vi "readMATFIle2.vi"(11 "selected path":path) -> (0 "dt2":dbl[](array[numeric]), 1 "Graph":cluster{dbl, dbl, "Magnitude":dbl[]}[](graph), 2 "Array":T2(array[cluster]), 3 "Title":string, 4 "npts":dbl, 5 "fsampling":dbl, 6 "tfun":dbl)   [LabVIEW 2024]
uses:
  Subs/miDataType.ctl
panel:
  out "text translated":string
  out "Left":string
  # "time chan    spect    sonogram"
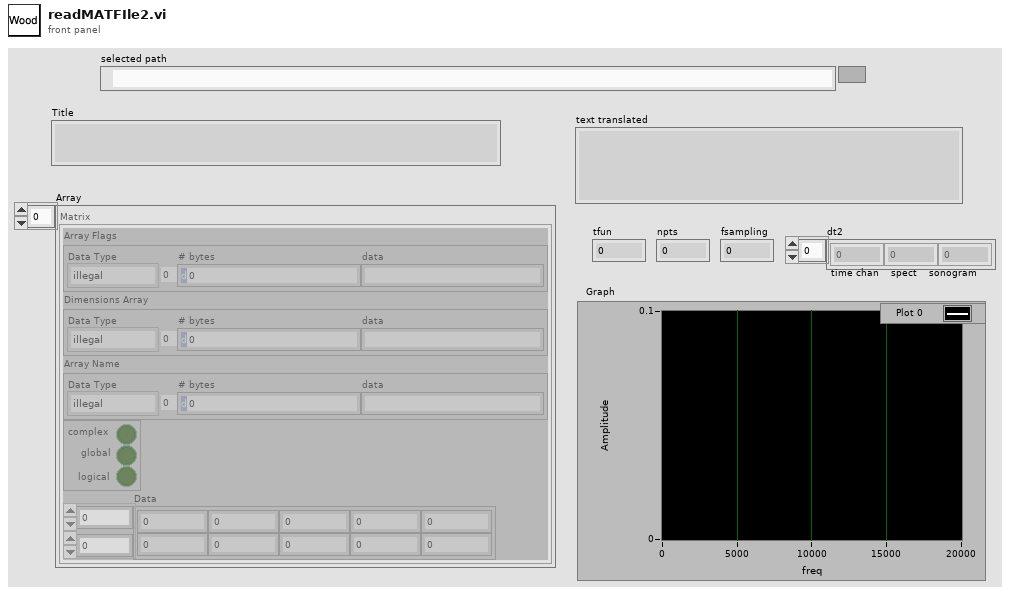
[diagram p1: front panel]
types:
  T1 = typedef "miDataType.ctl" = enum16{"illegal", "miINT8", "miUINT8", "miINT16", "miUINT16", "miINT32", "miUINT32", "miSINGLE", "--", "miDOUBLE", "---", "----", "miINT64", "miUINT64", "miMATRIX", "miCOMPRESSED", "miUTF8", "miUTF16", "miUTF32", "udefined"}
  T2 = cluster{"Array Flags":cluster{"Data Type":T1, "# bytes":u32, "data":string}, "Dimensions Array":cluster{"Data Type":T1, "# bytes":u32, "data":string}, "Array Name":cluster{"Data Type":T1, "# bytes":u32, "data":string}, cluster{"complex":bool, "global":bool, "logical":bool}, "Data":dbl[][]}[]
  T3 = enum16{"big-endian, network order", "native, host order", "little-endian"}
  T4 = cluster{"Data Type":T1, "# bytes":u32, "data":string}
  T5 = cluster{"Array Flags":cluster{"Data Type":T1, "# bytes":u32, "data":string}, "Dimensions Array":cluster{"Data Type":T1, "# bytes":u32, "data":string}, "Array Name":cluster{"Data Type":T1, "# bytes":u32, "data":string}, cluster{"complex":bool, "global":bool, "logical":bool}, "Data":dbl[][]}
  T6 = cluster{"TFRFHeader":cluster{"index":u32, "Xr":dbl, "Yr":dbl, "XActual":dbl, "YActual":dbl}, "Frequency Axis":cluster{"Hz Resolution":dbl, "Start Freq":dbl, "End Freq":dbl}, "TSingleArray":cluster{"fComplex":u32, "fLength":dbl, "a[2]":dbl, "fConditionCheck":dbl, "Precision":dbl, "MtxVecVersion":dbl, "SizeOf(TSample)":dbl, "Tag":dbl, "MtxVecFileCode":dbl, "a[9]":dbl, "a[10]":dbl}, "caption":string}
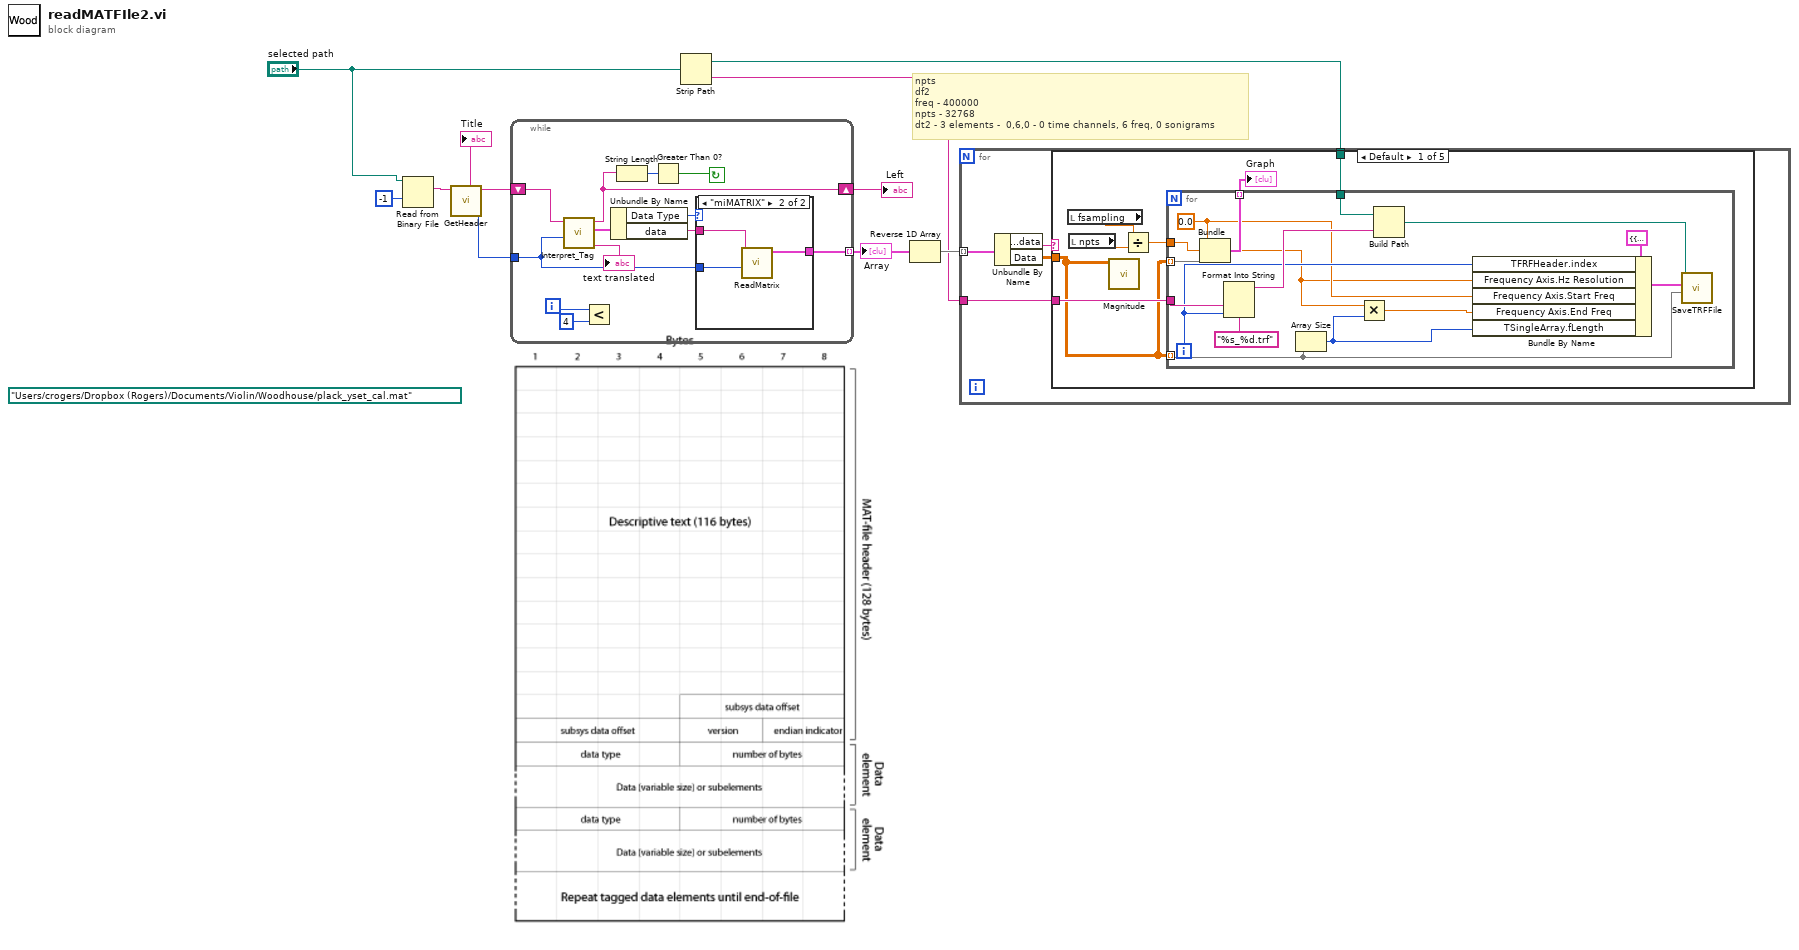
[diagram p0: block diagram]
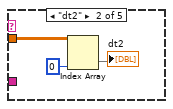
[diagram p3: hidden frame]
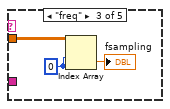
[diagram p4: hidden frame]
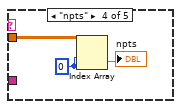
[diagram p5: hidden frame]
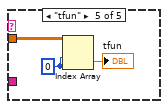
[diagram p6: hidden frame]
diagram:
  (unwired) path "/Users/crogers/Dropbox (Rogers)/Documents/Violin/Woodhouse/plack_yset_cal.mat" ("file (use dialog)")
  # "npts\ndf2\nfreq - 400000\nnpts - 32768\ndt2 - 3 elements -  0,6,0 - 0 time channels, 6 freq, 0 sonigrams"
  n1 = Read from Binary File(10:-1 ("count (1)"), 11:"selected path") -> (2:w10:string)  [unwired: 4 in, 3 out]
  n2 = call "GetHeader.vi"("String in"=w10) -> ("Endian"=w8:T3, "String out"=w7:string, "Title"=→"Title":string)  [unwired: 8 in]
  n3 = while {
    shift-right: [w17] -> w4
    shift-left: w7 -> [w22]
    tunnel: [w20] -> w6 mode=indexing
    tunnel: w8 -> [w19]
    i -> [w15]
    stop <- w12 continue-if-true
    n4 = call "Interpret_Tag.vi"("byte order"=w19, "String in"=w22) -> ("text translated"=→"text translated":string, "Tag"=w23:T4, "String out"=w17:string)  [unwired: 7 in]
    n5 = Less?(x=w15, y=4) -> ()  [unwired: 1 out]
    n6 = Unbundle By Name(w23) -> ("Data Type"=w18:T1, "data"=w21:string)
    n7 = String Length(string=w17) -> (length=w16:i32)
    n8 = Greater Than 0?(x=w16) -> (x > 0?=w12:bool)
    n9 = case shown="\"miMATRIX\"" w18 {
      tunnel: w21 -> [_ w26]
      tunnel: [_ w24] -> w20
      tunnel: w19 -> [_ w25]
      frame Default {
      }
      frame "miMATRIX" {
        n10 = call "ReadMatrix.vi"("byte order"=w25, "String in"=w26) -> ("Matrix"=w24:T5)  [unwired: 6 in, 3 out]
      }
    }
  }
  "Array" <- w6
  "Left" <- w4
  n11 = Strip Path(path="selected path") -> (stripped path=w2:path, name=w3:string)
  n12 = Reverse 1D Array(array=w6) -> (reversed array=w5:T2)
  n13 = for {
    tunnel: w5 -> [w31] mode=indexing
    tunnel: w3 -> [w28]
    tunnel: w2 -> [w27]
    n14 = Unbundle By Name(w31) -> ("Array Name.data"=w30:string, "Data"=w29:dbl[][])
    n15 = case shown="Default" w30 {
      tunnel: w29 -> [w32 w54 w57 w60 w63]
      tunnel: w28 -> [w35 _ _ _ _]
      tunnel: w27 -> [w34 _ _ _ _]
      frame Default {
        n16 = local read "fsampling"() -> (w38:dbl)
        n17 = local read "npts"() -> (w37:dbl)
        n18 = call "Magnitude.vi"("Data in"=w32) -> ()  [unwired: 8 in, 3 out]
        n19 = Divide(x=w38, y=w37) -> (x/y=w36:dbl)
        n20 = for {
          tunnel: w36 -> [w41]
          tunnel: w32 -> [w40] mode=indexing
          tunnel: w35 -> [w46]
          tunnel: w34 -> [w48]
          tunnel: [w43] -> w33 mode=indexing
          tunnel: w32 -> [w39] mode=indexing
          i -> [w44]
          w42 = 0.0
          n21 = Bundle(w42, w41, "Data"=w40) -> (w43:cluster{dbl, dbl, "Data":dbl[]})  [unwired: 1 in]
          n22 = Format Into String(format string="%s_%d.trf", w46, w44) -> (resulting string=w47:string)  [unwired: 2 in, 1 out]
          n23 = Array Size(array=w39) -> (size(s)=w51:i32)
          n24 = Multiply(x=w41, y=w51) -> (x*y=w52:dbl)
          n25 = Build Path(base path=w48, name or relative path=w47) -> (appended path=w45:path)
          n26 = Bundle By Name(cluster=T6 {"TFRFHeader"={"index"=11, "Xr"=0.0, "Yr"=0.0, "XActual"=0.0, "YActual"=0.0}, "Frequency Axis"={"Hz Resolution"=0.732421875, "Start Freq"=199.951171875, "End Freq"=9999.755859375}, "TSingleArray"={"fComplex"=1, "fLength"=13381.0, "a[2]"=0.0, "fConditionCheck"=1.0, "Precision"=0.0, "MtxVecVersion"=420.0, "SizeOf(TSample)"=8.0, "Tag"=0.0, "MtxVecFileCode"=64019.0, "a[9]"=0.0, "a[10]"=0.0}, "caption"="\u0000\u0000\u0000\u0000"} ("Header Info"), "TFRFHeader.index"=w44, "Frequency Axis.Hz Resolution"=w41, "Frequency Axis.Start Freq"=w42, "Frequency Axis.End Freq"=w52, "TSingleArray.fLength"=w51) -> (w49:T6)
          n27 = call "SaveTRFFile.vi"("Y"=w39, "Header Info"=w49, "trf file in"=w45) -> ()  [unwired: 7 in, 2 out]
        }
        "Graph" <- w33
      }
      frame "dt2" {
        n28 = Index Array(array=w54, index (col)=0 ("index (row)")) -> (element=→"dt2":dbl[])  [unwired: 1 in]
      }
      frame "freq" {
        w58 = 0 ("index (row)")
        n29 = Index Array(array=w57, index (row)=w58, index (col)=w58) -> (element=→"fsampling":dbl)
      }
      frame "npts" {
        w61 = 0 ("index (row)")
        n30 = Index Array(array=w60, index (row)=w61, index (col)=w61) -> (element=→"npts":dbl)
      }
      frame "tfun" {
        w64 = 0 ("index (row)")
        n31 = Index Array(array=w63, index (row)=w64, index (col)=w64) -> (element=→"tfun":dbl)
      }
    }
  }
